vi "Get Val BOOL.vi"(8 "error in (no error)":errorcluster, 10 "Lookup String":string, 11 "PropertyObject in":refnum<class "PropertyObject.lvclass">) -> (0 "error out":errorcluster, 2 "Value":bool, 3 "PropertyObject out":refnum<class "PropertyObject.lvclass">)   [LabVIEW 2020, in "TSnax.lvlib" / "PropertyObject.lvclass"]
uses:
  PropertyObject.lvclass
  PropertyObject.lvclass/PropertyObject.ctl
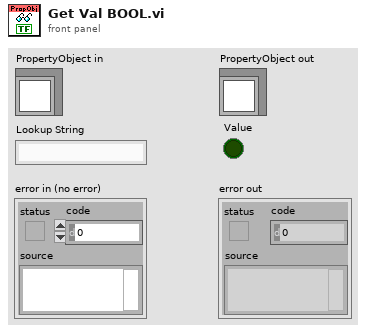
[diagram p1: front panel]
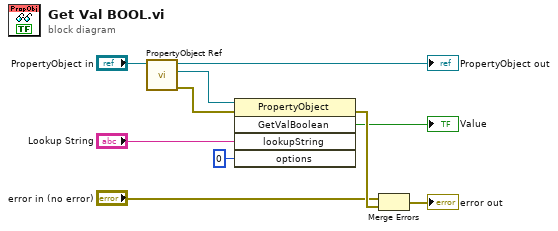
[diagram p0: block diagram]
diagram:
  n1 = call "PropertyObject Ref.vi"("PropertyObject in"="PropertyObject in") -> ("error out"=w5:errorcluster, "PropertyObject"=w6:refnum<k7>, "PropertyObject out"=→"PropertyObject out":refnum<class "PropertyObject.lvclass">)  [unwired: 8 in]
  n2 = invoke class="PropertyObject" method="GetValBoolean"(reference=w6, error in=w5, "lookupString"="Lookup String", "options"=0) -> (error out=w10:errorcluster, "GetValBoolean"=→"Value":bool)  [unwired: 1 in, 3 out]
  n3 = Merge Errors("error in (no error)", w10) -> (→"error out":errorcluster)
